vi "readJsonConfig.vi"(8 "error in":errorcluster, 11 "jsonConfig":string) -> (0 "error out":errorcluster={"status"=TRUE, "code"=0, "source"=""}, 1 "DAQmx Cluster Out":T2 {"ai DAQmx Cluster"."input terminal configuration" items=["Default"=-1, "RSE"=10083, "NRSE"=10078, "Differential"=10106, "Pseudodifferential"=12529]; "bc DAQmx Cluster"."Scaling Information"."electrical units" items=["Volts/Volt"=15896, "mVolts/Volt"=15897]; "bc DAQmx Cluster"."Scaling Information"."physical units" items=["Newtons"=15875, "Pounds"=15876, "kgf"=15877]; "bc DAQmx Cluster"."Bridge Information"."bridge configuration" items=["Full Bridge"=10182, "Half Bridge"=10187, "Quarter Bridge"=10270]; "bc DAQmx Cluster"."Bridge Information"."voltage excitation source" items=["Internal"=10200, "External"=10167]; "tc DAQmx Cluster"."Thermocouple Type" items=["J"=10072, "K"=10073, "N"=10077, "R"=10082, "S"=10085, "T"=10086, "B"=10047, "E"=10055]; "tc DAQmx Cluster"."Units" items=["Deg C"=10143, "Deg F"=10144, "Kelvins"=10325, "Deg R"=10145, "From Custom Scale"=10065]}, 2 "StreamCluster":T1={"DAQ"={"ManagmentRate_Hz"=1, "StreamRate_Hz"=50, "refDesArray"=[], "StreamRate_ms"=20, "ManagmentRate_ms"=1000}, "Modules"=[]}, 3 "Calibration Configuration Out":T3)   [LabVIEW 2024]
uses:
  Configuration/DAQmx Configuration.ctl
  Configuration/Calibration Configuration.ctl
  Control/StreamCluster_TypeDef.ctl
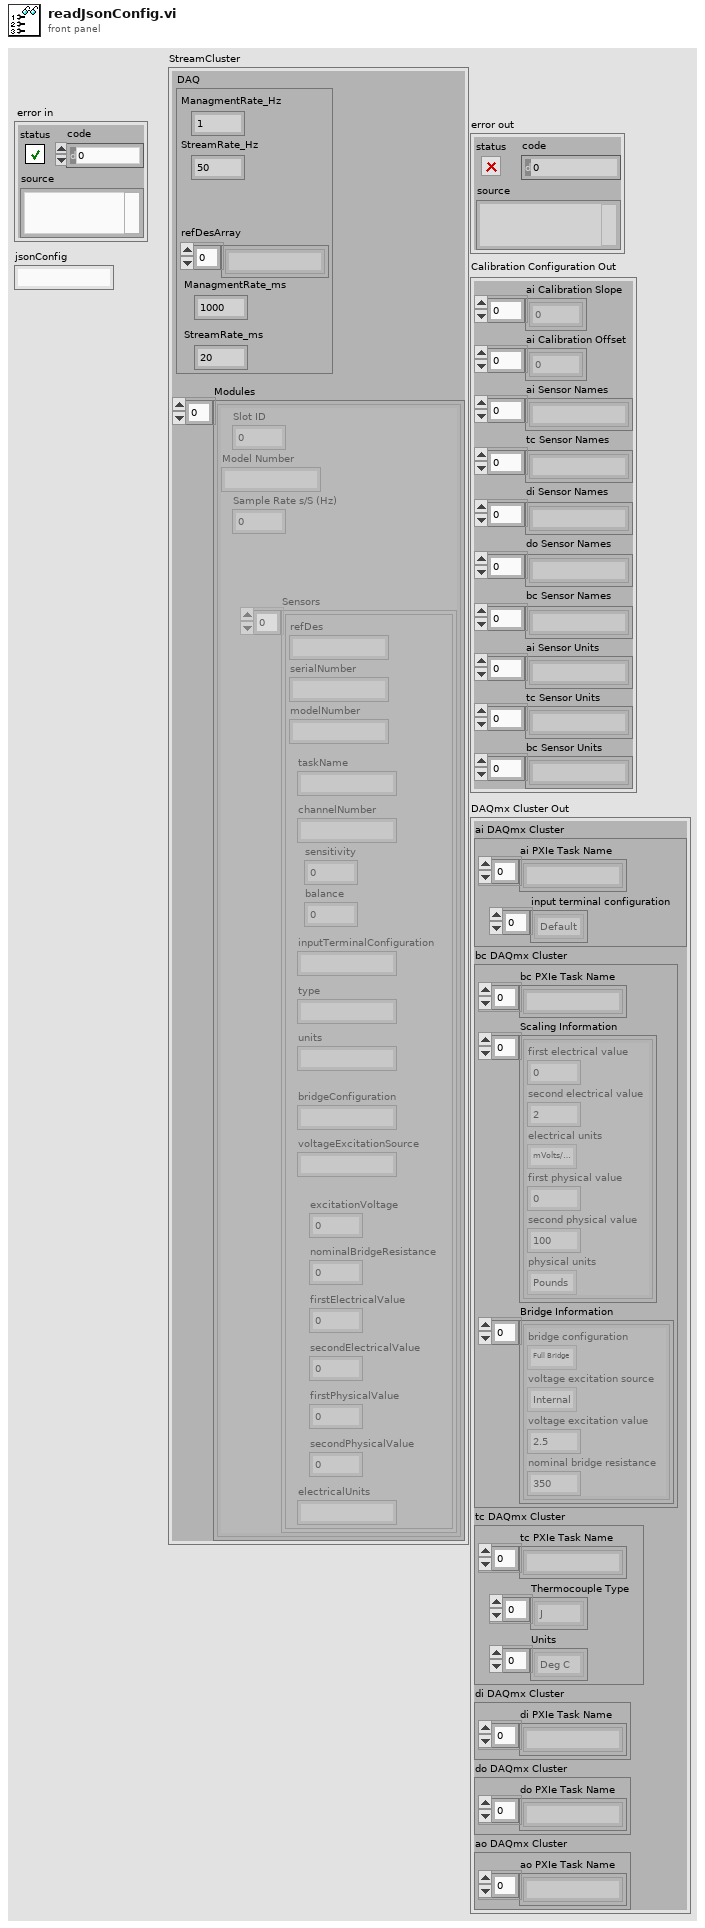
[diagram p1: front panel]
types:
  T1 = typedef "StreamCluster_TypeDef.ctl" = cluster{"DAQ":cluster{"ManagmentRate_Hz":i32, "StreamRate_Hz":i32, "refDesArray":string[], "StreamRate_ms":i32, "ManagmentRate_ms":i32}, "Modules":cluster{"Slot ID":i32, "Model Number":string, "Sample Rate s/S (Hz)":dbl, "Sensors":cluster{"refDes":string, "serialNumber":string, "modelNumber":string, "units":string, "balance":dbl, "sensitivity":dbl, "type":string, "inputTerminalConfiguration":string, "channelNumber":string, "taskName":string, "bridgeConfiguration":string, "excitationVoltage":dbl, "voltageExcitationSource":string, "nominalBridgeResistance":dbl, "firstElectricalValue":dbl, "secondElectricalValue":dbl, "firstPhysicalValue":dbl, "secondPhysicalValue":dbl, "electricalUnits":string}[]}[]}
  T2 = typedef "DAQmx Configuration.ctl" = cluster{"ai DAQmx Cluster":cluster{"ai PXIe Task Name":string[], "input terminal configuration":i32[]}, "bc DAQmx Cluster":cluster{"bc PXIe Task Name":string[], "Scaling Information":cluster{"first electrical value":dbl, "second electrical value":dbl, "electrical units":i32, "first physical value":dbl, "second physical value":dbl, "physical units":i32}[], "Bridge Information":cluster{"bridge configuration":i32, "voltage excitation source":i32, "voltage excitation value":dbl, "nominal bridge resistance":dbl}[]}, "tc DAQmx Cluster":cluster{"tc PXIe Task Name":string[], "Thermocouple Type":i32[], "Units":i32[]}, "di DAQmx Cluster":cluster{"di PXIe Task Name":string[]}, "do DAQmx Cluster":cluster{"do PXIe Task Name":string[]}, "ao DAQmx Cluster":cluster{"ao PXIe Task Name":string[]}}
  T3 = typedef "Calibration Configuration.ctl" = cluster{"ai Calibration Slope":dbl[], "ai Calibration Offset":dbl[], "ai Sensor Names ":string[], "tc Sensor Names":string[], "di Sensor Names":string[], "do Sensor Names":string[], "bc Sensor Names":string[], "ai Sensor Units":string[], "tc Sensor Units":string[], "bc Sensor Units":string[]}
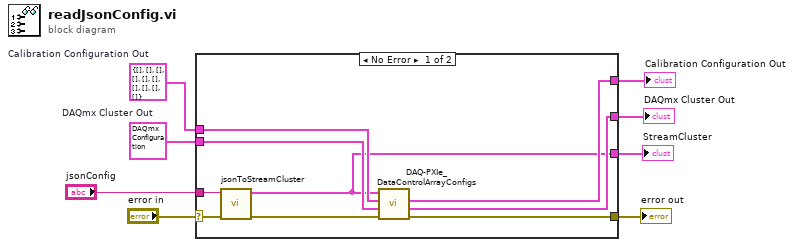
[diagram p0: block diagram]
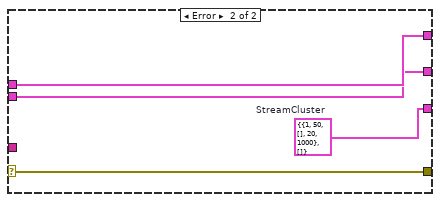
[diagram p2: hidden frame]
diagram:
  w4 = T3 {"ai Calibration Slope"=[], "ai Calibration Offset"=[], "ai Sensor Names "=[], "tc Sensor Names"=[], "di Sensor Names"=[], "do Sensor Names"=[], "bc Sensor Names"=[], "ai Sensor Units"=[], "tc Sensor Units"=[], "bc Sensor Units"=[]}  # Calibration Configuration Out
  w3 = T2 {"ai DAQmx Cluster"={"ai PXIe Task Name"=[], "input terminal configuration"=[]}, "bc DAQmx Cluster"={"bc PXIe Task Name"=[], "Scaling Information"=[], "Bridge Information"=[]}, "tc DAQmx Cluster"={"tc PXIe Task Name"=[], "Thermocouple Type"=[], "Units"=[]}, "di DAQmx Cluster"={"di PXIe Task Name"=[]}, "do DAQmx Cluster"={"do PXIe Task Name"=[]}, "ao DAQmx Cluster"={"ao PXIe Task Name"=[]}}  # DAQmx Cluster Out
  n1 = case shown="No Error" "error in" {
    selector: "error in" -> [w12 w21]
    tunnel: [w17 w21] -> w7
    tunnel: [w14 w20] -> w6
    tunnel: [w13 w19] -> w5
    tunnel: w4 -> [w16 w20]
    tunnel: w3 -> [w15 w19]
    tunnel: "jsonConfig" -> [w10 _]
    tunnel: [w9 w18] -> w1
    frame No Error {
      n2 = call "jsonToStreamCluster.vi"("error in"=w12, "jsonConfig"=w10) -> ("error out"=w11:errorcluster, "StreamCluster"=w9:T1)  [unwired: 8 in]
      n3 = call "DAQ-PXIe_DataControlArrayConfigs.vi"("error in"=w11, "DAQmx Cluster In"=w15, "Calibration Configuration In"=w16, "StreamCluster_TypeDef"=w9) -> ("error out"=w17:errorcluster, "DAQmx Cluster Out"=w13:T2, "Calibration Configuration Out"=w14:T3)  [unwired: 5 in]
    }
    frame Error {
      w18 = T1 {"DAQ"={"ManagmentRate_Hz"=1, "StreamRate_Hz"=50, "refDesArray"=[], "StreamRate_ms"=20, "ManagmentRate_ms"=1000}, "Modules"=[]}  # StreamCluster
    }
  }
  "error out" <- w7
  "Calibration Configuration Out" <- w6
  "DAQmx Cluster Out" <- w5
  "StreamCluster" <- w1
